vi "StreamBus.Do.vi"(10 "State Variables":T2, 11 "gRPCid":T1) -> (2 "State Variables out":T2)   [LabVIEW 2025, in "xnet_can_bus_monitor_api_server_do.lvlib"]
uses:
  xnet_can_bus_monitor_api_server_do.lvlib
  Types/MainProcess.StateVariables.ctl
  Types/XNET.InitialSettings.ctl
  xnet_can_bus_monitor_api_server/RPC Messages/ni_xnet_can_bm_api_ConnectSettings.ctl
  xnet_can_bus_monitor_api_server/RPC Messages/ni_xnet_can_bm_api_CanMode.ctl
  xnet_can_bus_monitor_api_server/RPC Messages/ni_xnet_can_bm_api_Termination.ctl
  xnet_can_bus_monitor_api_server/RPC Messages/ni_xnet_can_bm_api_FdIsoMode.ctl
  xnet_can_bus_monitor_api_server/RPC Messages/ni_xnet_can_bm_api_FilterInfo.ctl
  xnet_can_bus_monitor_api_server/RPC Messages/ni_xnet_can_bm_api_DirectionFilter.ctl
  xnet_can_bus_monitor_api_server/RPC Messages/ni_xnet_can_bm_api_FrameFilter.ctl
  Types/StreamProcess.Refs.ctl
  Types/StreamProcess.VIRef.ctl
  <vilib>/gRPC/LabVIEW gRPC Library/Shared/grpcId.ctl
  Types/StreamProcess.InputRefs.ctl
  xnet_can_bus_monitor_api_server/RPC Messages/ni_xnet_can_bm_api_StreamBusReply.ctl
  xnet_can_bus_monitor_api_server/RPC Messages/ni_xnet_can_bm_api_CanCommState.ctl
  xnet_can_bus_monitor_api_server/RPC Messages/ni_xnet_can_bm_api_CommState.ctl
  xnet_can_bus_monitor_api_server/RPC Messages/ni_xnet_can_bm_api_LastCommError.ctl
  xnet_can_bus_monitor_api_server/RPC Messages/ni_xnet_can_bm_api_Frame.ctl
  xnet_can_bus_monitor_api_server/RPC Messages/ni_xnet_can_bm_api_ErrorInfo.ctl
  SubVIs/StreamProcess.Main.vi
  <vilib>/gRPC/LabVIEW gRPC Library/grpc-lvsupport-release.lvlib
  xnet_can_bus_monitor_api_server/xnet_can_bus_monitor_api_server.lvlib
  xnet_can_bus_monitor_api_server/RPC Service/NI_XNET_CAN_Bus_Monitor_API/NI_XNET_CAN_Bus_Monitor_API.lvclass
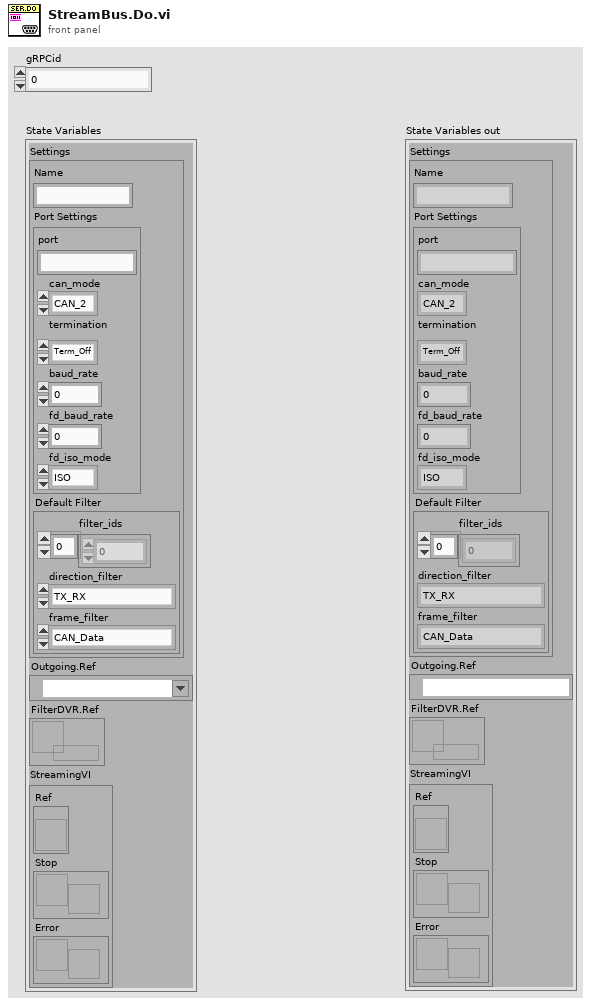
[diagram p1: front panel]
types:
  T1 = typedef "grpc-lvsupport-release.lvlib/grpcId.ctl" = u64
  T2 = typedef "xnet_can_bus_monitor_api_server_do.lvlib/MainProcess.StateVariables.ctl" = cluster{"Settings":T3, "Outgoing.Ref":refnum<k21>, "FilterDVR.Ref":refnum<data-value>, "StreamingVI":T11}
  T3 = typedef "xnet_can_bus_monitor_api_server_do.lvlib/XNET.InitialSettings.ctl" = cluster{"Name":string, "Port Settings":T4, "Default Filter":T8}
  T4 = typedef "xnet_can_bus_monitor_api_server.lvlib/ni_xnet_can_bm_api_ConnectSettings.ctl" = cluster{"port":string, "can_mode":T5, "termination":T6, "baud_rate":u64, "fd_baud_rate":u64, "fd_iso_mode":T7}
  T5 = typedef "xnet_can_bus_monitor_api_server.lvlib/ni_xnet_can_bm_api_CanMode.ctl" = enum32{"CAN_2", "CAN_FD", "CAN_FD_BRS"}
  T6 = typedef "xnet_can_bus_monitor_api_server.lvlib/ni_xnet_can_bm_api_Termination.ctl" = enum32{"Term_Off", "Term_On"}
  T7 = typedef "xnet_can_bus_monitor_api_server.lvlib/ni_xnet_can_bm_api_FdIsoMode.ctl" = enum32{"ISO", "Non_ISO", "ISO_Legacy"}
  T8 = typedef "xnet_can_bus_monitor_api_server.lvlib/ni_xnet_can_bm_api_FilterInfo.ctl" = cluster{"filter_ids":u32[], "direction_filter":T9, "frame_filter":T10}
  T9 = typedef "xnet_can_bus_monitor_api_server.lvlib/ni_xnet_can_bm_api_DirectionFilter.ctl" = enum32{"TX_RX", "RX", "TX"}
  T10 = typedef "xnet_can_bus_monitor_api_server.lvlib/ni_xnet_can_bm_api_FrameFilter.ctl" = enum32{"CAN_Data", "CAN_Remote", "CAN_Bus_Error", "CAN_2_Data", "CAN_FD_Data", "CAN_FD_BRS_Data", "J1939_Data", "Delay", "Log_Trigger", "Start_Trigger", "All"}
  T11 = typedef "xnet_can_bus_monitor_api_server_do.lvlib/StreamProcess.Refs.ctl" = cluster{"Ref":T12, "Stop":refnum<notifier>, "Error":refnum<notifier>}
  T12 = typedef "xnet_can_bus_monitor_api_server_do.lvlib/StreamProcess.VIRef.ctl" = refnum<vi>
  T13 = typedef "xnet_can_bus_monitor_api_server_do.lvlib/StreamProcess.InputRefs.ctl" = cluster{"ReportError":refnum<notifier>, "CheckStop":refnum<notifier>, "gRPCid":T1}
  T14 = typedef "xnet_can_bus_monitor_api_server.lvlib/ni_xnet_can_bm_api_StreamBusReply.ctl" = cluster{"can_comm_state":T15, "frame":T18[], "error":T19}
  T15 = typedef "xnet_can_bus_monitor_api_server.lvlib/ni_xnet_can_bm_api_CanCommState.ctl" = cluster{"fault_code":i32, "fault":bool, "comm_state":T16, "last_comm_error":T17, "receive_error_counter":u32, "transmit_error_counter":u32, "transceiver_error":bool, "sleep":bool}
  T16 = typedef "xnet_can_bus_monitor_api_server.lvlib/ni_xnet_can_bm_api_CommState.ctl" = enum32{"Error_Active", "Error_Passive", "Bus_Off", "Init"}
  T17 = typedef "xnet_can_bus_monitor_api_server.lvlib/ni_xnet_can_bm_api_LastCommError.ctl" = enum32{"None", "Stuff", "Form", "ACK", "Bit1", "Bit0", "CRC"}
  T18 = typedef "xnet_can_bus_monitor_api_server.lvlib/ni_xnet_can_bm_api_Frame.ctl" = cluster{"timestamp":dbl, "payload":u8[], "identifier":u32, "frame_type":u32, "extended":bool, "echo":bool}
  T19 = typedef "xnet_can_bus_monitor_api_server.lvlib/ni_xnet_can_bm_api_ErrorInfo.ctl" = errorcluster
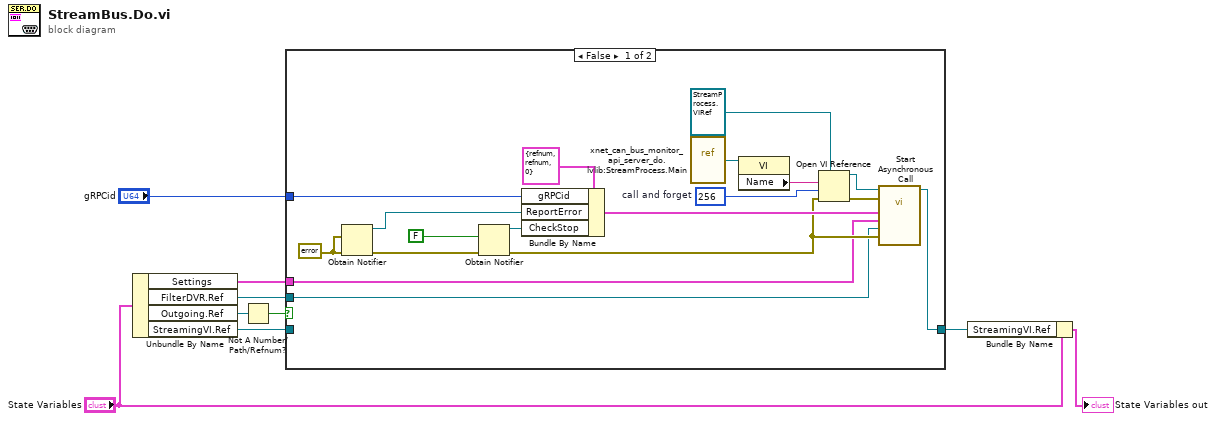
[diagram p0: block diagram]
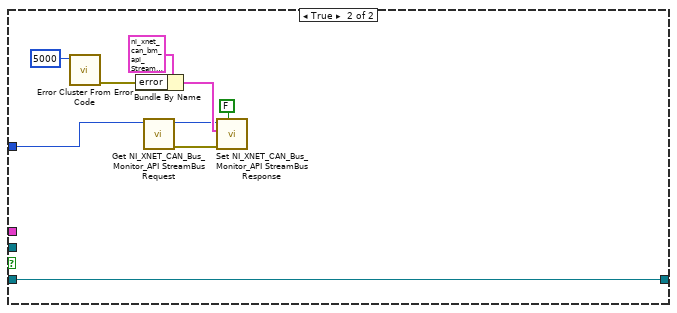
[diagram p2: hidden frame]
diagram:
  n1 = Unbundle By Name("State Variables") -> ("Settings"=w3:T3, "FilterDVR.Ref"=w4:refnum<data-value>, "Outgoing.Ref"=w5:refnum<k21>, "StreamingVI.Ref"=w6:T12)
  n2 = Not A Number/Path/Refnum?(number/path/refnum=w5) -> (NaN/Path/Refnum?=w2:bool)
  n3 = case shown="False" w2 {
    tunnel: "gRPCid" -> [w17 w33]
    tunnel: [w13 w28] -> w9
    tunnel: w3 -> [w11 _]
    tunnel: w4 -> [w10 _]
    tunnel: w6 -> [_ w28]
    frame False {
      w18 = errorcluster {"status"=FALSE, "code"=0, "source"=""} ("error in (no error)")
      w26 = 256  # call and forget
      n4 = Obtain Notifier(notification data type=w18, error in (no error)=w18) -> (notifier out=w21:refnum<notifier>, error out=w23:errorcluster)  [unwired: 2 in, 1 out]
      n5 = Obtain Notifier(notification data type=FALSE, error in (no error)=w23) -> (notifier out=w20:refnum<notifier>, error out=w14:errorcluster)  [unwired: 2 in, 1 out]
      n6 = Bundle By Name(cluster=T13 {"ReportError"=refnum, "CheckStop"=refnum, "gRPCid"=0}, "gRPCid"=w17, "ReportError"=w21, "CheckStop"=w20) -> (w15:T13)
      n7 = vi-ref "xnet_can_bus_monitor_api_server_do.lvlib:StreamProcess.Main.vi"() -> (w16:refnum<vi>)
      n8 = property class="VI"(reference=w16) -> ("Name"=w24:string)  [unwired: 1 in, 2 out]
      n9 = Open VI Reference(type specifier VI Refnum (for type only)=T12 refnum, vi path=w24, options=w26, error in (no error)=w14) -> (vi reference=w25:T12, error out=w27:errorcluster)  [unwired: 2 in]
      n10 = call-by-ref "Start Asynchronous Call"(reference=w25, error in=w27, 8:"error in (no error)"=w14, "FilterDVR.Ref"=w10, "Settings"=w11, "Refs"=w15) -> (reference out=w13:T12)  [unwired: 7 in, 2 out]
    }
    frame True {
      n11 = call <vilib>:"Error Cluster From Error Code.vi"("error code (0)"=5000) -> ("error out"=w29:errorcluster)  [unwired: 8 in]
      n12 = Bundle By Name(cluster=T14 {"can_comm_state"={"fault_code"=0, "fault"=FALSE, "comm_state"=enum."Error_Active", "last_comm_error"=enum."None", "receive_error_counter"=0, "transmit_error_counter"=0, "transceiver_error"=FALSE, "sleep"=FALSE}, "frame"=[], "error"={"status"=FALSE, "code"=0, "source"=""}} ("Message Data"), "error"=w29) -> (w34:T14)
      n13 = call "Get NI_XNET_CAN_Bus_Monitor_API StreamBus Request.vi"("gRPCid"=w33) -> ("error out"=w31:errorcluster, "gRPCid out"=w32:T1)  [unwired: 8 in, 1 out]
      n14 = call "Set NI_XNET_CAN_Bus_Monitor_API StreamBus Response.vi"("Streaming? (F)"=FALSE, "error in (no error)"=w31, "Message Data"=w34, "gRPCid in"=w32) -> ()  [unwired: 7 in, 1 out]
    }
  }
  n15 = Bundle By Name(cluster="State Variables", "StreamingVI.Ref"=w9) -> (→"State Variables out":T2)
